vi "acquireMeasurement.vi"(0 "startWL (nm)":dbl=1530.0 format="%.2f", 1 "numScans (1)":u32=1, 3 "Type of Measurement":u16(ring)=1 items=["Reflection", "Transmission"], 5 "endWL (nm)":dbl=1540.0 format="%.2f", 7 "Cont Scan?":bool, 9 "dutLength (m)":dbl=3.0 format="%.2f", 11 "error in (no error)":errorcluster) -> (4 "reAlign?":bool, 6 "reCalibrate?":bool, 8 "Cancelled?":bool, 10 "WL Cal Failed":bool, 14 "NoValidScansAcquired?":bool, 15 "error out":errorcluster)   [LabVIEW 2024]
uses:
  Matrices.ctl
  OVA_Global_Vars.vi
  Program Files (x86)/Luna Technologies/OVA 5000 v5.14.2/data/OVA32.dll
panel:
  out "numScansAttempted":u32
  out "valid Scans":u32
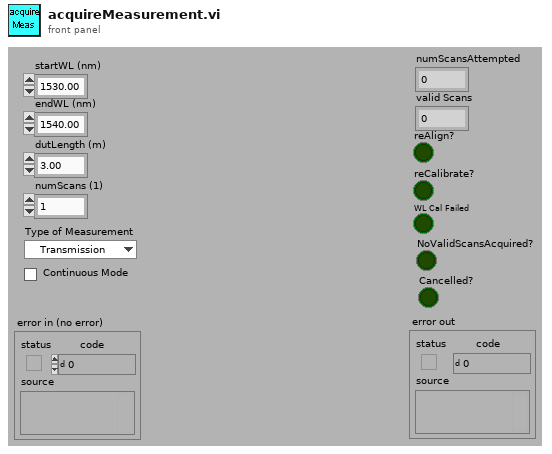
[diagram p1: front panel]
types:
  T1 = typedef "Matrices.ctl" = enum16{"Meas A", "Meas B", "Meas C", "Transfer", "Source", "Detector", "Temporary", "Temporary2", "Temporary3"}
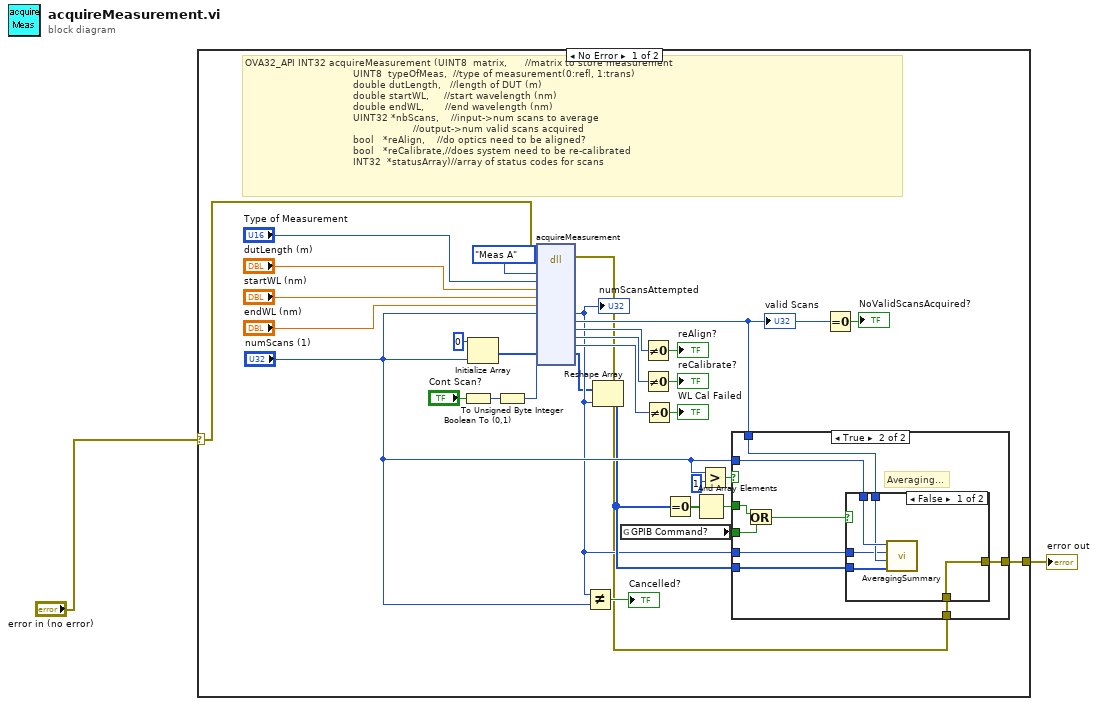
[diagram p0: block diagram]
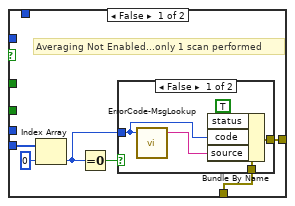
[diagram p2: hidden frame]
diagram:
  n1 = case shown="No Error" "error in (no error)" {
    selector: "error in (no error)" -> [w4 w61]
    tunnel: [w33 w61] -> w2
    frame No Error {
      # "OVA32_API INT32 acquireMeasurement (UINT8  matrix,      //matrix to store measurement\n                                    UINT8  typeOfMeas,  //type of measurement(0:refl, 1:trans)\n                                    double dutLength,   //length of DUT (m)\n                                    double startWL,     //start wavelength (nm)\n                                    double endWL,       //end wavelength (nm)\n                                    UINT32 *nbScans,    //input->num scans to average\n                                                        //output->num valid scans acquired\n                                    bool   *reAlign,    //do optics need to be aligned?\n                                    bool   *reCalibrate,//does system need to be re-calibrated\n                                    INT32  *statusArray)//array of status codes for scans"
      n2 = Boolean To (0,1)(Boolean="Cont Scan?") -> (0, 1=w8:i16)
      n3 = Initialize Array(0, "numScans (1)") -> (w12:i32[])
      n4 = To Unsigned Byte Integer(number=w8) -> (unsigned 8bit integer=w7:u8)
      n5 = dll-call lib="C:/Program Files (x86)/Luna Technologies/OVA 5000 v5.14.2/data/OVA32.dll" fn="acquireMeasurement" label="acquireMeasurement()"(error in=w4, "matrix"=Matrices."Meas A" ("Matrix"), "typeOfMeasurement"="Type of Measurement", "dutLength"="dutLength (m)", "startWL"="startWL (nm)", "endWL"="endWL (nm)", "numScans"="numScans (1)", "statusArray"=w12, "continous"=w7) -> (error out=w3:errorcluster, "numScans"=w10:u32, "validScans"=w16:u32, "reAlign"=w15:u8, "reCalibrate"=w14:u8, "wlCalFailed"=w13:u8, "statusArray"=w6:i32[])  [unwired: 13 in, 1 out]
      "valid Scans" <- w16
      "numScansAttempted" <- w10
      n6 = Not Equal?(x=w10, y="numScans (1)") -> (x != y?=→"Cancelled?":bool)
      n7 = Reshape Array(w6, w10) -> (w11:i32[])
      n8 = global read "OVA_Global_Vars.vi" "GPIB Command?"() -> (w5:bool)
      n9 = Not Equal To 0?(x=w15) -> (x != 0?=→"reAlign?":bool)
      n10 = Not Equal To 0?(x=w14) -> (x != 0?=→"reCalibrate?":bool)
      n11 = Not Equal To 0?(x=w13) -> (x != 0?=→"WL Cal Failed":bool)
      n12 = Equal To 0?(x=w11) -> (x = 0?=w18:bool[])
      n13 = And Array Elements(Boolean array=w18) -> (logical AND=w17:bool)
      n14 = Greater?(x="numScans (1)", y=u32 1) -> (0:w20:bool)
      n15 = case shown="True" w20 {
        tunnel: w11 -> [w38 w54]
        tunnel: "numScans (1)" -> [_ w50]
        tunnel: w16 -> [_ w53]
        tunnel: w3 -> [w37 w52]
        tunnel: [w34 w51] -> w33
        tunnel: w17 -> [_ w48]
        tunnel: w10 -> [_ w49]
        tunnel: w5 -> [_ w47]
        frame False {
          # "Averaging Not Enabled...only 1 scan performed"
          n16 = Index Array(array=w38, index=0 ("Index")) -> (element=w35:i32)
          n17 = Equal To 0?(x=w35) -> (x = 0?=w36:bool)
          n18 = case shown="False" w36 {
            tunnel: [w40 w45] -> w34
            tunnel: w37 -> [w44 w45]
            tunnel: w35 -> [w41 _]
            frame False {
              n19 = call "ErrorCode-MsgLookup.vi"("DLL Return Code"=w41) -> ("Error String"=w43:string)  [unwired: 2 in, 2 out]
              n20 = Bundle By Name(cluster=w44, "status"=TRUE, "code"=w41, "source"=w43) -> (w40:errorcluster)
            }
            frame True {
            }
          }
        }
        frame True {
          # "Averaging..."
          n21 = Or(x=w48, y=w47) -> (x .or. y?=w46:bool)
          n22 = case shown="False" w46 {
            tunnel: w54 -> [w58 _]
            tunnel: w53 -> [w56 _]
            tunnel: w50 -> [w57 _]
            tunnel: [w59 w60] -> w51
            tunnel: w52 -> [w59 w60]
            tunnel: w49 -> [w55 _]
            frame False {
              n23 = call "AveragingSummary.vi"("statusArray"=w58, "Number of Valid Scans"=w56, "Number of Scans Attempted"=w55, "Number of Scans Requested"=w57) -> ()  [unwired: 6 in]
            }
            frame True {
              # "No scans failed...everything OK"
            }
          }
        }
      }
      n24 = Equal To 0?(x=w16) -> (x = 0?=→"NoValidScansAcquired?":bool)
    }
    frame Error {
    }
  }
  "error out" <- w2
